vi "Set CompactSubObj.vi"(8 "error in":errorcluster, 10 "CompactSubObj":u8 format="%02x", 11 "Object Entry in":refnum<class "Object Entry.lvclass">) -> (0 "error out":errorcluster, 3 "Object Entry out":refnum<class "Object Entry.lvclass">)   [LabVIEW 2020, in "CANopen.lvlib" / "Object Entry.lvclass"]
uses:
  Object Entry.lvclass
  Object Entry.lvclass/Object Entry.ctl
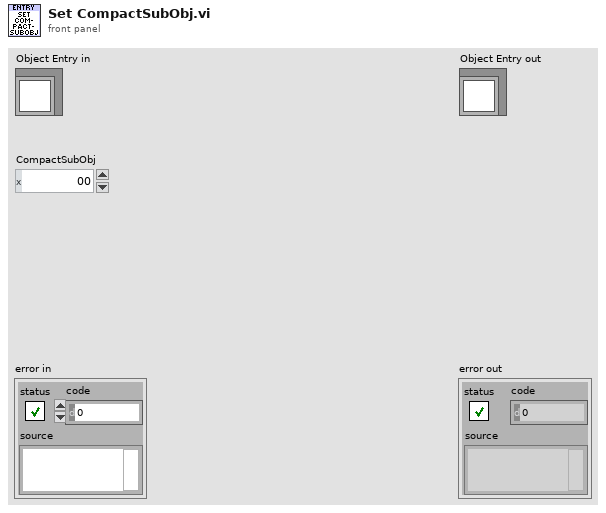
[diagram p1: front panel]
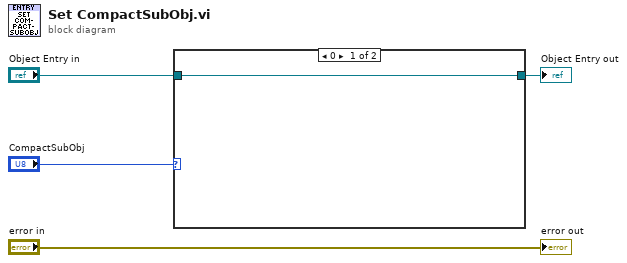
[diagram p0: block diagram]
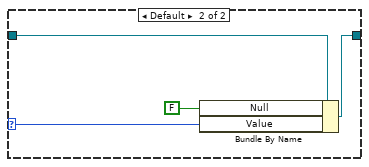
[diagram p2: hidden frame]
diagram:
  n1 = case shown="0" "CompactSubObj" {
    selector: "CompactSubObj" -> [_ w7]
    tunnel: "Object Entry in" -> [w5 w9]
    tunnel: [w5 w8] -> w3
    frame 0 {
    }
    frame Default {
      n2 = Bundle By Name(cluster=w9, "Null"=FALSE ("CompactSubObj.Null"), "Value"=w7) -> (w8:refnum<class "Object Entry.lvclass">)
    }
  }
  "Object Entry out" <- w3
  "error out" <- "error in"
